vi "Integration Test Launcher.vi"() -> ()   [LabVIEW 2020]
doc: "<License>\nCopyright © 2017 Composed Systems, LLC | All rights reserved\nwww.composed.io\n\nAuthor: Ethan Stern <ethan.stern@composed.io>\n\nThis software is provided \"AS IS\" WITHOUT WARRANTIES, either express or implied, AND IS FOR EDUCATIONAL PURPOSES ONLY.\n</License>"
uses:
  BasicChartBinding/BasicChartBinding.lvclass
  BasicTerminalBinding/BasicTerminalBinding.lvclass
  MultiSubscriber/MultiSubscriber.lvclass
  <vilib>/ActorFramework/Actor/Actor.lvclass
  ConcreteViewModel/ConcreteViewModel.lvclass
  Source/ViewManager/LeftListboxViewManager/LeftListboxViewManager.lvclass
  Source/ViewManager/TabbedViewManager/TabbedViewManager.lvclass
  Source/ViewManager/QuadViewManager/QuadViewManager.lvclass
  ActorAutoRegistrationView/EventHandlingActor.lvclass
  modules/mva-viewable/Source/IViewModel/IViewModel/IViewModel.lvclass
  modules/mva-viewable/Source/IViewable/IViewable Messages/Open Front Panel Msg/Open Front Panel Msg.lvclass
  modules/mva-viewable/Source/IViewable/IViewable/View Position Enum.ctl
  modules/mva-viewable/Source/IViewable/IViewable/IViewable.lvclass
  modules/mva-core/Source/IModel/IModel/IModel.lvclass
  <vilib>/ActorFramework/Message Enqueuer/Message Priority.ctl
  <vilib>/ActorFramework/Message Enqueuer/Message Enqueuer.lvclass
  ConcreteModel/ConcreteModel.lvclass
  ValueChangeEventProducer/ValueChangeEventProducer.lvclass
  Source/ViewManager/BoundViewManager/BoundViewManager.lvclass
  TreeActor/TreeActor.lvclass
  MCListboxActor/MCListboxActor.lvclass
  TestApplicationStyle/TestApplicationStyle.lvclass
  C:/Program Files/National Instruments/LabVIEW 2020/vi.lib/ActorFramework/Actor/Actor.lvclass
  52c60252-50fc-4a03-94af-d5c5c5d06c7f.vi
  modules/mva-viewable/Source/IViewable/IViewable Messages/Set Minimum Panel Size Msg/Set Minimum Panel Size Msg.lvclass
  <vilib>/Utility/miscctls.llb/LVPointTypeDef.ctl
  10e8937e-8001-4ee2-ad38-642db9692e9b.vi
  modules/mva-core/Source/MonitoredMediator/MonitoredMediator/MonitoredMediator.lvclass
  Source/BusMonitor/ListboxBusMonitor/ListboxBusMonitor/ListboxBusMonitor.lvclass
  modules/mva-core/Source/Mediator/Mediator/Mediator.lvclass
  modules/mva-viewable/Source/IViewManager/IViewManager/IViewManager.lvclass
panel:
  in  "中介监控":bool
  in  "订阅数量":i32=10
  in  "视图":i32=10
  out "error out":errorcluster
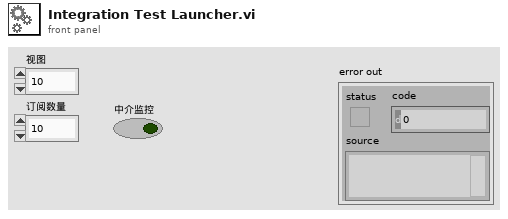
[diagram p1: front panel]
types:
  T1 = typedef "LVPointTypeDef.ctl" = cluster{"Horizontal":i16, "Vertical":i16}
  T2 = typedef "Actor Framework.lvlib/Message Enqueuer.lvclass/Message Priority.ctl" = enum16{"Low", "Normal", "High"}
  T3 = typedef "MVA Framework.lvlib/IViewable.lvlib/IViewable.lvclass/View Position Enum.ctl" = enum16{"Centered", "Maximized", "Minimized", "Custom", "Unchanged"}
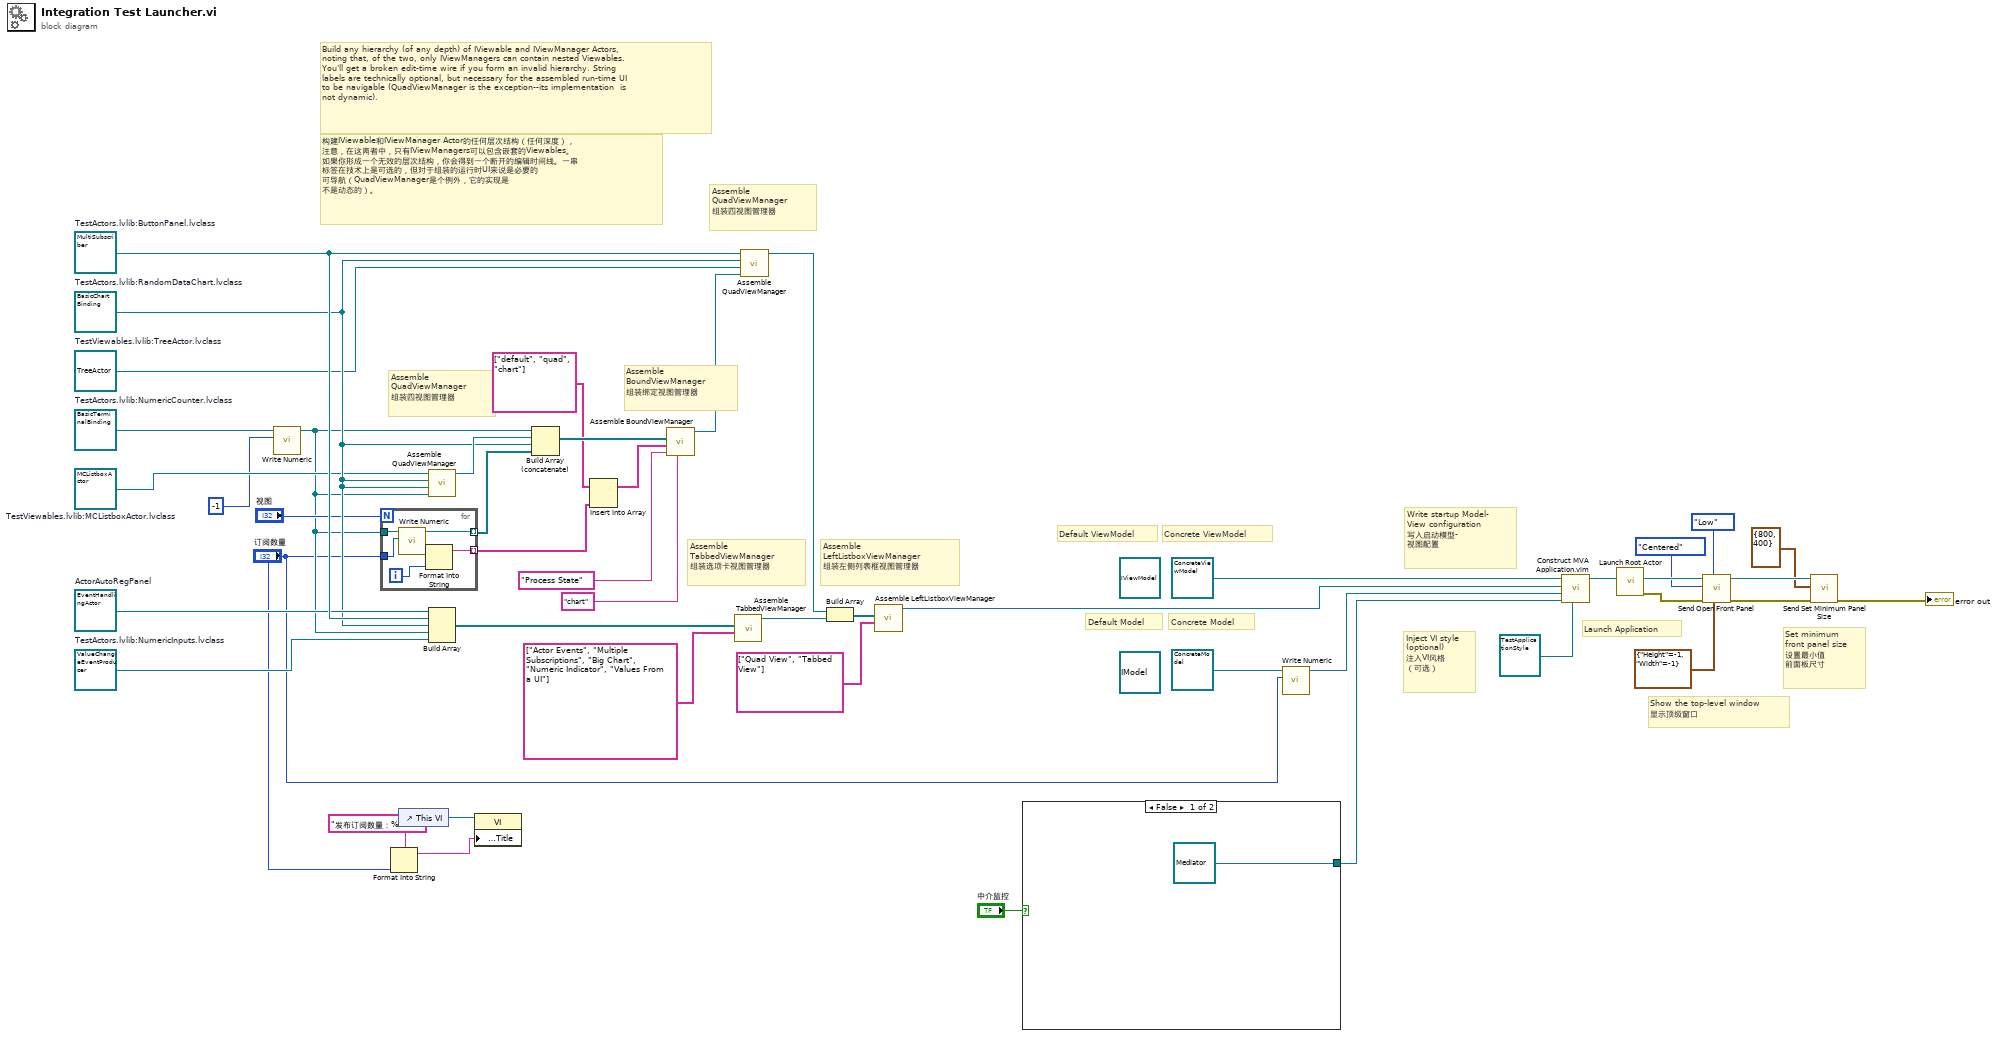
[diagram p0: block diagram]
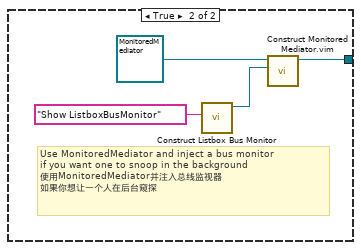
[diagram p2: hidden frame]
diagram:
  w23 = refnum<class "MCListboxActor.lvclass"> refnum  # TestViewables.lvlib:MCListboxActor.lvclass
  w24 = refnum<class "TreeActor.lvclass"> refnum  # TestViewables.lvlib:TreeActor.lvclass
  (unwired) refnum<class "IModel.lvclass"> refnum ("IModel.lvlib:IModel.lvclass")
  (unwired) refnum<class "IViewModel.lvclass"> refnum ("IController.lvlib:IController.lvclass")
  w36 = refnum<class "EventHandlingActor.lvclass"> refnum  # ActorAutoRegPanel
  w38 = refnum<class "ValueChangeEventProducer.lvclass"> refnum  # TestActors.lvlib:NumericInputs.lvclass
  w39 = refnum<class "MultiSubscriber.lvclass"> refnum  # TestActors.lvlib:ButtonPanel.lvclass
  w10 = refnum<class "BasicTerminalBinding.lvclass"> refnum  # TestActors.lvlib:NumericCounter.lvclass
  w25 = refnum<class "BasicChartBinding.lvclass"> refnum  # TestActors.lvlib:RandomDataChart.lvclass
  # "Assemble\nQuadViewManager\n组装四视图管理器"
  # "构建IViewable和IViewManager Actor的任何层次结构（任何深度），\n注意，在这两者中，只有IViewManagers可以包含嵌套的Viewables。\n如果你形成一个无效的层次结构，你会得到一个断开的编辑时间线。一串\n标签在技术上是可选的，但对于组装的运行时UI来说是必要的\n可导航（QuadViewManager是个例外，它的实现是\n不是动态的）。"
  # "Set minimum\nfront panel size\n设置最小值\n前面板尺寸"
  # "Inject VI style\n(optional)\n注入VI风格\n（可选）"
  # "Assemble\nBoundViewManager\n组装绑定视图管理器"
  # "Assemble\nQuadViewManager\n组装四视图管理器"
  # "Assemble\nLeftListboxViewManager\n组装左侧列表框视图管理器"
  # "Assemble\nTabbedViewManager\n组装选项卡视图管理器"
  # "Show the top-level window\n显示顶级窗口"
  # "Concrete Model"
  # "Default Model"
  # "Default ViewModel"
  # "Concrete ViewModel"
  # "Launch Application"
  # "Write startup Model-\nView configuration\n写入启动模型-\n视图配置"
  # "Build any hierarchy (of any depth) of IViewable and IViewManager Actors,\nnoting that, of the two, only IViewManagers can contain nested Viewables.\nYou'll get a broken edit-time wire if you form an invalid hierarchy. String\nlabels are technically optional, but necessary for the assembled run-time UI\nto be navigable (QuadViewManager is the exception--its implementation  is\nnot dynamic)."
  n1 = call-dynamic "Write Numeric.vi"("Numeric"=-1, "BasicTerminalBinding in"=w10) -> ("BasicTerminalBinding out"=w9:refnum<class "BasicTerminalBinding.lvclass">)  [unwired: 8 in, 1 out]
  n2 = for {
    N: "视图" -> [_]
    tunnel: w9 -> [w50]
    tunnel: [w49] -> w15 mode=indexing
    tunnel: [w51] -> w12 mode=indexing
    tunnel: "订阅数量" -> [w47]
    i -> [w48]
    n3 = call-dynamic "Write Numeric.vi"("Numeric"=w47, "BasicTerminalBinding in"=w50) -> ("BasicTerminalBinding out"=w49:refnum<class "BasicTerminalBinding.lvclass">)  [unwired: 8 in, 1 out]
    n4 = Format Into String(w48) -> (resulting string=w51:string)  [unwired: 3 in, 1 out]
  }
  n5 = Format Into String(format string="发布订阅数量：%d", "订阅数量") -> (resulting string=w5:string)  [unwired: 2 in, 1 out]
  n6 = control-ref of="This VI"() -> (w7:refnum<vi>)
  n7 = call "Assemble QuadViewManager.vi"("Bottom-Right View"=w9, "Bottom-Left View"=w25, "Top-Right View"=w25, "Top-Left View"=w23) -> ("QuadViewManager out"=w28:refnum<class "QuadViewManager.lvclass">)  [unwired: 7 in]
  n8 = Build Array(w36, w39, w25, w9, w38) -> (w45:refnum<class "IViewable.lvclass">[])
  n9 = property class="VI"(reference=w7, "Front Panel.Title"=w5) -> ()  [unwired: 1 in, 2 out]
  n10 = Build Array (concatenate)(w9, w28, w25, w15) -> (w27:refnum<class "IViewable.lvclass">[])
  n11 = Insert Into Array(array=string[] ["default", "quad", "chart"] ("Insertion Names"), new element=w12) -> (w14:string[])  [unwired: 1 in]
  n12 = call "Assemble BoundViewManager.vi"("Startup View Name (\"\"=None)"="chart" ("Startup View Name (\"\"=None)"), "Selector String Name"="Process State", "Viewable Names"=w14, "Bound Viewables"=w27) -> ("BoundViewManager Out"=w29:refnum<class "BoundViewManager.lvclass">)  [unwired: 7 in]
  n13 = call "Assemble TabbedViewManager.vi"("View Names"=string[] ["Actor Events", "Multiple Subscriptions", "Big Chart", "Numeric Indicator", "Values From a UI"] ("View Labels"), "Views"=w45) -> ("TabbedViewManager Out"=w42:refnum<class "TabbedViewManager.lvclass">)  [unwired: 9 in]
  n14 = call "Assemble QuadViewManager.vi"("Bottom-Right View"=w29, "Bottom-Left View"=w24, "Top-Right View"=w25, "Top-Left View"=w39) -> ("QuadViewManager out"=w37:refnum<class "QuadViewManager.lvclass">)  [unwired: 7 in]
  n15 = Build Array(w37, w42) -> (w44:refnum<class "IViewManager.lvclass">[])
  n16 = call "Assemble LeftListboxViewManager.vi"("View Names"=string[] ["Quad View", "Tabbed View"] ("View Labels"), "Views"=w44) -> ("LeftListboxViewManager Out"=w43:refnum<class "LeftListboxViewManager.lvclass">)  [unwired: 9 in]
  n17 = case shown="False" "中介监控" {
    tunnel: [refnum<class "Mediator.lvclass"> refnum ("MVA Framework.lvlib:Mediator.lvlib:Mediator.lvclass") w55] -> w18
    frame False {
    }
    frame True {
      # "Use MonitoredMediator and inject a bus monitor\nif you want one to snoop in the background\n使用MonitoredMediator并注入总线监视器\n如果你想让一个人在后台窥探"
      n18 = call "Construct Listbox Bus Monitor.vi"("Show Panel Boolean Name"="Show ListboxBusMonitor") -> ("ListboxBusMonitor out"=w54:refnum<class "ListboxBusMonitor.lvclass">)  [unwired: 10 in]
      n19 = call "Construct Monitored Mediator.vim"("Startup Bus Monitor(s)"=w54, "MonitoredMediator in"=refnum<class "MonitoredMediator.lvclass"> refnum ("MonitoredMediator.lvlib:MonitoredMediator.lvclass")) -> ("MonitoredMediator out"=w55:refnum<class "MonitoredMediator.lvclass">)  [unwired: 9 in]
    }
  }
  n20 = call-dynamic "Write Numeric.vi"("Numeric"="订阅数量", "ConcreteModel in"=refnum<class "ConcreteModel.lvclass"> refnum ("TopLevelApplication.lvlib:ConcreteModel.lvclass")) -> ("ConcreteModel out"=w2:refnum<class "ConcreteModel.lvclass">)  [unwired: 8 in, 1 out]
  n21 = call "Construct MVA Application.vim"("Application Style"=refnum<class "TestApplicationStyle.lvclass"> refnum ("TestApplicationStyle.lvclass"), "Mediator Type"=w18, "Model Type"=w2, "Startup View Configuration"=w43, "IViewModel In"=refnum<class "ConcreteViewModel.lvclass"> refnum ("TopLevelApplication.lvlib:TopLevelApplication.lvclass")) -> ("IViewModel Out"=w46:refnum<class "ConcreteViewModel.lvclass">)  [unwired: 6 in]
  n22 = call <vilib>:"Launch Root Actor.vi"("Actor"=w46) -> ("error out"=w33:errorcluster, "Actor's Enqueuer"=w35:refnum<class "Message Enqueuer.lvclass">)  [unwired: 9 in]
  n23 = call "Send Open Front Panel.vi"("Custom Window Size"=cluster{"Height":i16, "Width":i16} {"Height"=-1, "Width"=-1} ("Custom Size"), "Message Priority (Normal)"=Message_Priority."Low", "error in (no error)"=w33, "Position"=View_Position_Enum."Centered", "Message Enqueuer"=w35) -> ("error out"=w34:errorcluster, "Message Enqueuer out"=w20:refnum<class "Message Enqueuer.lvclass">)  [unwired: 5 in]
  n24 = call "Send Set Minimum Panel Size.vi"("error in (no error)"=w34, "Minimum Size"=T1 {"Horizontal"=800, "Vertical"=400}, "Message Enqueuer"=w20) -> ("error out"=→"error out":errorcluster)  [unwired: 7 in, 1 out]
